vi "RSNRPZ Set Led Mode.vi"(8 "error in (no error)":errorcluster, 9 "Mode (User Settings)":u32(ring)=1 items=["User Settings"=1, "Sensor Function"=2], 10 "Channel (1)":i32=1, 11 "VISA session":refnum<visa-resource-name> caption="VISA resource name") -> (0 "error out":errorcluster, 3 "dup VISA session":refnum<visa-resource-name> caption="VISA resource name")   [LabVIEW 2010]
doc: "This VI sets the led mode.\n\nRemote-control command(s):\nSYST:LED:MODE"
uses:
  rsnrpz_32.dll
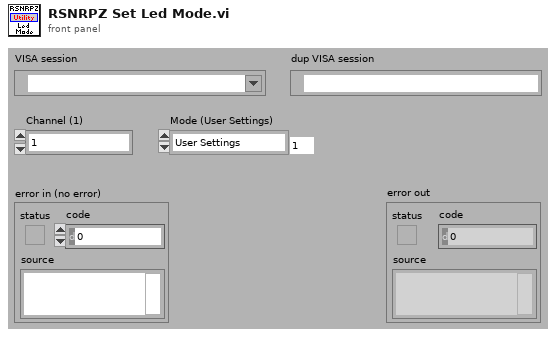
[diagram p1: front panel]
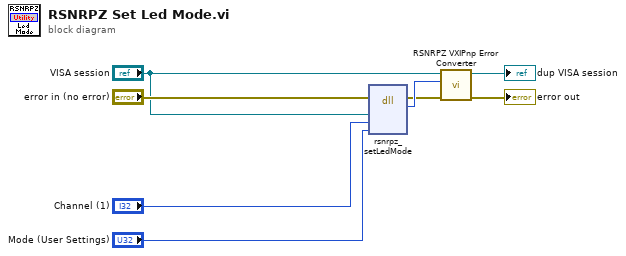
[diagram p0: block diagram]
diagram:
  n1 = dll-call lib="rsnrpz_32.dll" fn="rsnrpz_setLedMode"(error in="error in (no error)", "Instrument Handle"="VISA session", "Channel"="Channel (1)", "Mode"="Mode (User Settings)") -> (error out=w5:errorcluster, w6:i32)  [unwired: 5 in, 1 out]
  n2 = call <instrlib>:"RSNRPZ VXIPnp Error Converter.vi"("error in"=w5, "VXIPnp error code"=w6, "VISA session"="VISA session") -> ("error out"=→"error out":errorcluster, "dup VISA session"=→"dup VISA session":refnum<visa-resource-name>)  [unwired: 7 in]
